vi "LoadCommParam.vi"(10 "section name":string) -> (2 "output cluster":T1)   [LabVIEW 2018]
uses:
  <vilib>/Utility/config.llb/Read Key (U32).vi
  <vilib>/Utility/config.llb/Read Key (String).vi
  <vilib>/Utility/config.llb/NI_LVConfig.lvlib
panel:
  out "error out":errorcluster
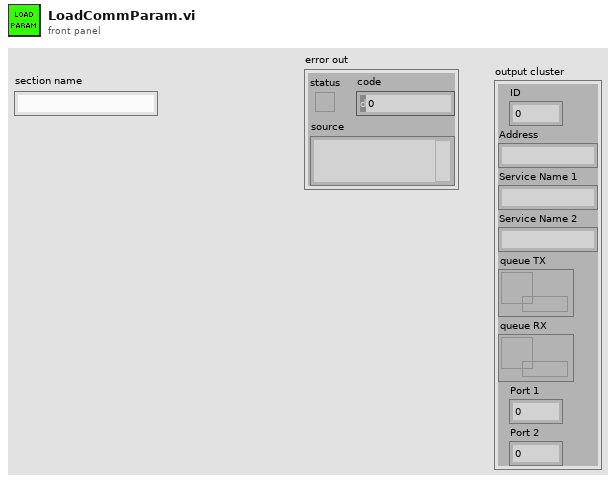
[diagram p1: front panel]
types:
  T1 = cluster{"ID":u32, "Address":string, "Service Name 1":string, "Service Name 2":string, "queue TX":refnum<queue>, "queue RX":refnum<queue>, "Port 1":u32, "Port 2":u32}
  T2 = typedef "NI_LVConfig.lvlib/Config Data RefNum.ctl" = refnum<k1>
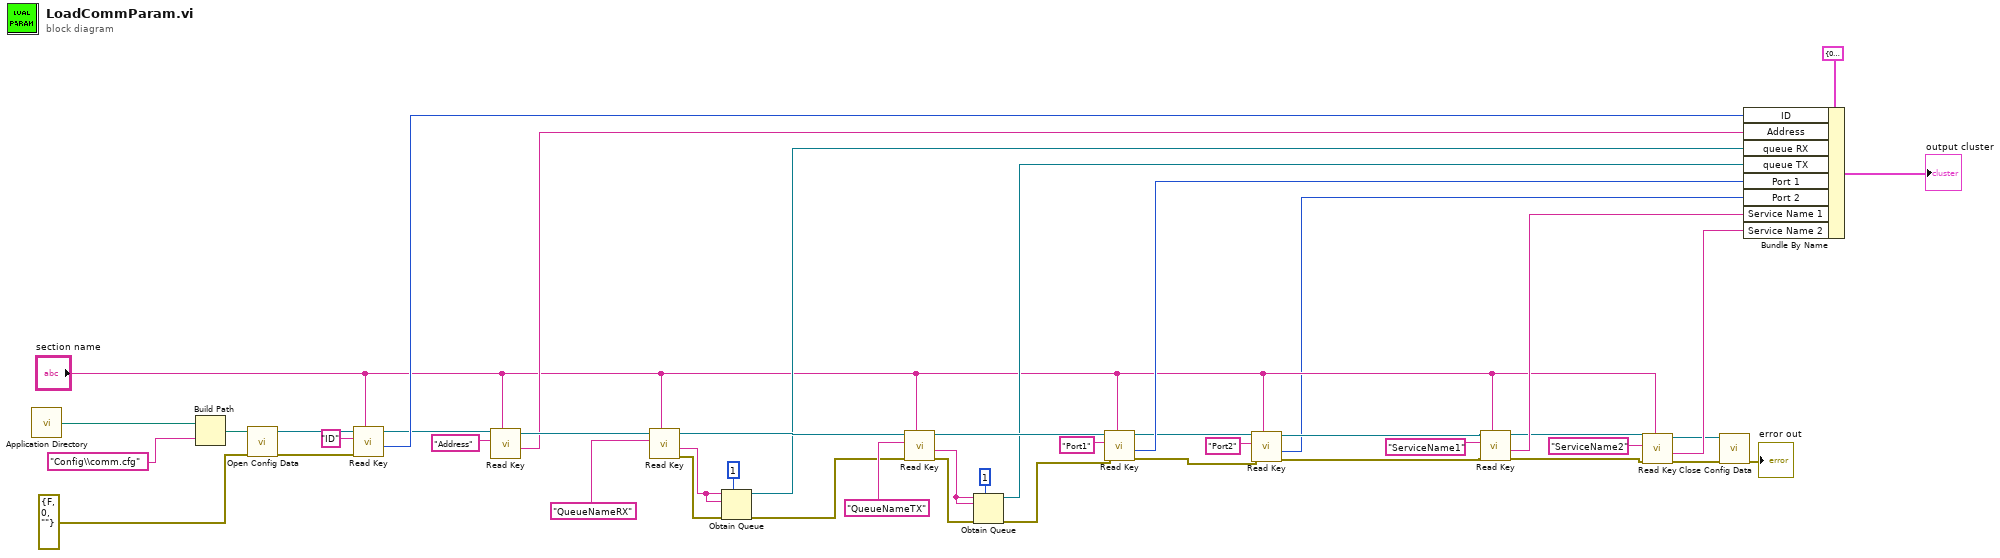
[diagram p0: block diagram]
diagram:
  n1 = call <vilib>:"Application Directory.vi"() -> ("Application Directory"=w1:path)
  n2 = Build Path(base path=w1, name or relative path="Config\\comm.cfg") -> (appended path=w46:path)
  n3 = call <vilib>:"Open Config Data.vi"("error in (no error)"=errorcluster {"status"=FALSE, "code"=0, "source"=""}, "configuration file path"=w46) -> ("error out"=w43:errorcluster, "refnum"=w45:T2)  [unwired: 7 in, 1 out]
  n4 = call-poly <vilib>:"Read Key.vi"("section"="section name", "error in (no error)"=w43, "key"="ID", "refnum"=w45) -> ("value"=w25:u32, "refnum out"=w18:T2)  [unwired: 4 in, 2 out]
  n5 = call-poly <vilib>:"Read Key.vi"("section"="section name", "key"="Address", "refnum"=w18) -> ("value"=w16:string, "refnum out"=w17:T2)  [unwired: 5 in, 2 out]
  n6 = call-poly <vilib>:"Read Key.vi"("section"="section name", "key"="QueueNameRX", "refnum"=w17) -> ("error out"=w34:errorcluster, "value"=w40:string, "refnum out"=w39:T2)  [unwired: 5 in, 1 out]
  n7 = Obtain Queue(max queue size (-1, unlimited)=1, name (unnamed)=w40, element data type=w40, error in (no error)=w34) -> (queue out=w24:refnum<queue>, error out=w33:errorcluster)  [unwired: 1 in, 1 out]
  n8 = call-poly <vilib>:"Read Key.vi"("section"="section name", "error in (no error)"=w33, "key"="QueueNameTX", "refnum"=w39) -> ("error out"=w32:errorcluster, "value"=w41:string, "refnum out"=w28:T2)  [unwired: 4 in, 1 out]
  n9 = Obtain Queue(max queue size (-1, unlimited)=1, name (unnamed)=w41, element data type=w41, error in (no error)=w32) -> (queue out=w23:refnum<queue>, error out=w29:errorcluster)  [unwired: 1 in, 1 out]
  n10 = call-poly <vilib>:"Read Key.vi"("section"="section name", "error in (no error)"=w29, "key"="Port1", "refnum"=w28) -> ("error out"=w7:errorcluster, "value"=w10:u32, "refnum out"=w5:T2)  [unwired: 4 in, 1 out]
  n11 = call-poly <vilib>:"Read Key.vi"("section"="section name", "error in (no error)"=w7, "key"="Port2", "refnum"=w5) -> ("error out"=w6:errorcluster, "value"=w2:u32, "refnum out"=w4:T2)  [unwired: 4 in, 1 out]
  n12 = call-poly <vilib>:"Read Key.vi"("section"="section name", "error in (no error)"=w6, "key"="ServiceName1", "refnum"=w4) -> ("error out"=w13:errorcluster, "value"=w22:string, "refnum out"=w15:T2)  [unwired: 4 in, 1 out]
  n13 = call-poly <vilib>:"Read Key.vi"("section"="section name", "error in (no error)"=w13, "key"="ServiceName2", "refnum"=w15) -> ("error out"=w12:errorcluster, "value"=w20:string, "refnum out"=w14:T2)  [unwired: 4 in, 1 out]
  n14 = call <vilib>:"Close Config Data.vi"("error in (no error)"=w12, "refnum"=w14) -> ("error out"=→"error out":errorcluster)  [unwired: 8 in, 1 out]
  n15 = Bundle By Name(cluster=T1 {"ID"=0, "Address"="", "Service Name 1"="", "Service Name 2"="", "queue TX"=refnum, "queue RX"=refnum, "Port 1"=0, "Port 2"=0} ("Comm Parameters"), "ID"=w25, "Address"=w16, "queue RX"=w24, "queue TX"=w23, "Port 1"=w10, "Port 2"=w2, "Service Name 1"=w22, "Service Name 2"=w20) -> (→"output cluster":T1)
